vi "WRP Get Detector Region.vi"(8 "error in (no error)":errorcluster) -> (0 "error out":errorcluster, 2 "function return":i32, 3 "value":T1)   [LabVIEW 2018, in "SesWrapper.lvlib"]
doc: "int STDCALL WRP_GetDetectorRegion(DetectorRegion *value);"
uses:
  SesWrapper.lvlib
  build/Debug/SESWrapper.dll
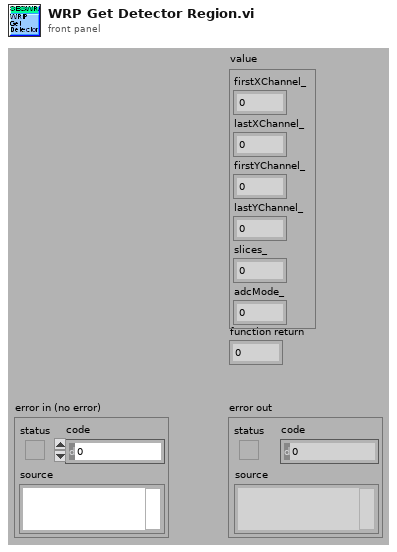
[diagram p1: front panel]
types:
  T1 = cluster{"firstXChannel_":i32, "lastXChannel_":i32, "firstYChannel_":i32, "lastYChannel_":i32, "slices_":i32, "adcMode_":u8}
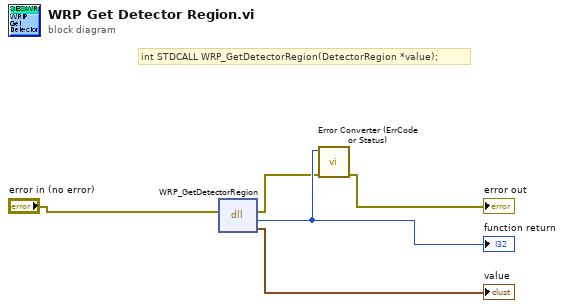
[diagram p0: block diagram]
diagram:
  # "int STDCALL WRP_GetDetectorRegion(DetectorRegion *value);"
  n1 = dll-call lib="C:/Development/svn/seswrapper-lib/build/Debug/SESWrapper.*" fn="WRP_GetDetectorRegion"(error in="error in (no error)") -> (error out=w2:errorcluster, w5:i32, "value"=→"value":T1)  [unwired: 3 in, 1 out]
  "function return" <- w5
  n2 = call "Error Converter (ErrCode or Status).vi"("error in (no error)"=w2, "error code"=w5) -> ("error out"=→"error out":errorcluster)  [unwired: 9 in]
